vi "Chroma_PowerSupply_ReadVolt.vi"(8 "错误输入（无错误）":errorcluster, 11 "VISA资源名称":refnum<visa-resource-name>) -> (0 "错误输出":errorcluster, 2 "Volt":dbl format="%.4f", 3 "VISA资源名称输出":refnum<visa-resource-name>)   [LabVIEW 8.6]
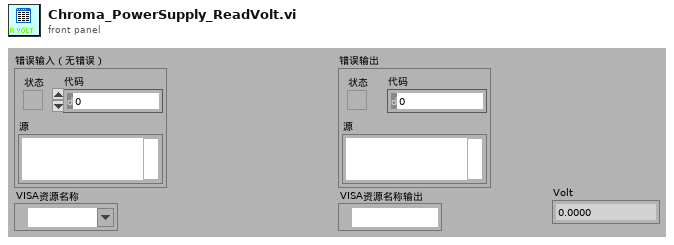
[diagram p1: front panel]
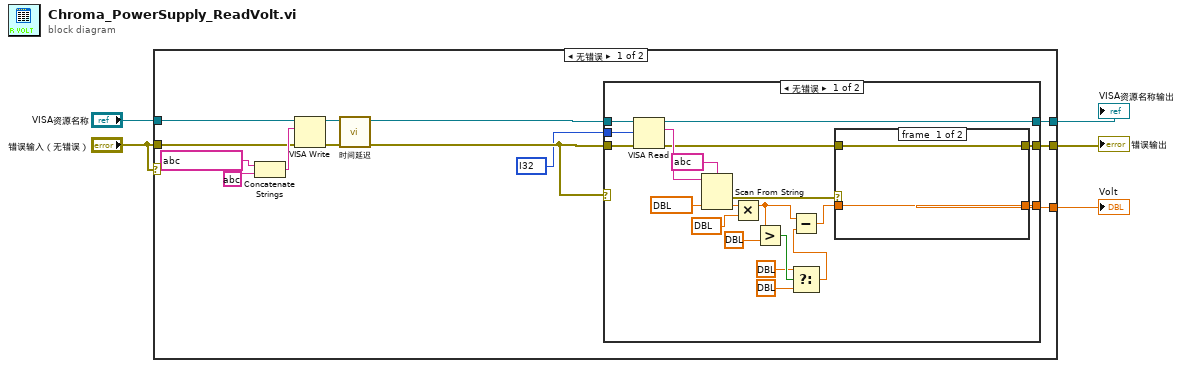
[diagram p0: block diagram]
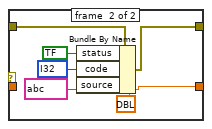
[diagram p2: hidden frame]
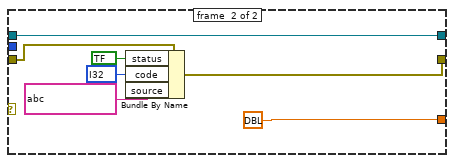
[diagram p3: hidden frame]
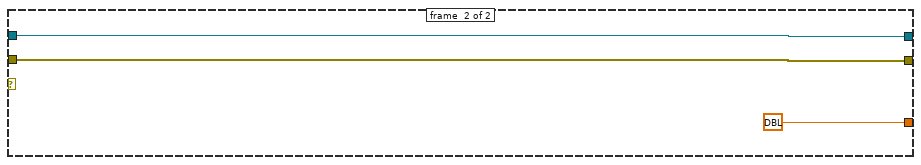
[diagram p4: hidden frame]
diagram:
  n1 = case shown="无错误" "错误输入（无错误）" {
    tunnel: "VISA资源名称" -> [w15 w55]
    tunnel: "错误输入（无错误）" -> [w14 w54]
    tunnel: [w12 w54] -> w4
    tunnel: [w11 w55] -> w3
    tunnel: [w9 dbl ? ("默认值 1")] -> w2
    frame #0 {
      n2 = Concatenate Strings(string ?, string ?) -> (w16:string)
      n3 = VISA Write(VISA resource name=w15, write buffer=w16, error in (no error)=w14) -> (VISA resource name out=w7:refnum<visa-resource-name>, error out=w13:errorcluster)  [unwired: 1 out]
      n4 = call "时间延迟"("error in (no error)"=w13) -> ("error out"=w8:errorcluster)  [unwired: 1 in, 9 out]
      n5 = case shown="无错误" w8 {
        tunnel: [w26 w50] -> w12
        tunnel: [w37 w52] -> w11
        tunnel: w7 -> [w36 w52]
        tunnel: w8 -> [w35 w49]
        tunnel: [w28 dbl ? ("默认值 1")] -> w9
        tunnel: i32 ? -> [w31 _]
        frame #0 {
          n6 = VISA Read(VISA resource name=w36, byte count=w31, error in (no error)=w35) -> (VISA resource name out=w37:refnum<visa-resource-name>, read buffer=w34:string, error out=w27:errorcluster)  [unwired: 1 out]
          n7 = Scan From String(format string=string ? ("格式字符串"), input string=w34, default 1=dbl ? ("默认值 1")) -> (error out=w30:errorcluster, output 1=w29:dbl)  [unwired: 2 in, 2 out]
          n8 = Multiply(x=w29, y=dbl ?) -> (x*y=w23:dbl)
          n9 = Greater?(x=w23, y=dbl ?) -> (0:w21:bool)
          n10 = Select(t=dbl ?, s=w21, f=dbl ?) -> (s? t:f=w18:dbl)
          n11 = Subtract(x=w23, y=w18) -> (x-y=w24:dbl)
          n12 = case shown="错误" w30 {
            tunnel: w24 -> [w39 _]
            tunnel: [w39 dbl ? ("默认值 1")] -> w28
            tunnel: w27 -> [w38 w41]
            tunnel: [w38 w42] -> w26
            frame #0 {
            }
            frame #1 {
              n13 = Bundle By Name(cluster=w41, "status"=bool ?, "code"=i32 ?, "source"=string ?) -> (w42:errorcluster)
            }
          }
        }
        frame #1 {
          n14 = Bundle By Name(cluster=w49, "status"=bool ?, "code"=i32 ?, "source"=string ?) -> (w50:errorcluster)
        }
      }
    }
    frame #1 {
    }
  }
  "错误输出" <- w4
  "VISA资源名称输出" <- w3
  "Volt" <- w2
